vi "Module-error.vi"(6 "Error":T1=enum."Not implemented", 8 "error in (no error)":errorcluster, 9 "Overwrite?":bool, 10 "Additional message":string) -> (0 "error out":errorcluster)   [LabVIEW 2013, in "MaterialCharacterization.lvlib" / "MC-SM1000.lvclass"]
uses:
  MC-SM1000.lvclass
  Custom-errors.ctl
  <vilib>/Utility/error.llb/DialogType.ctl
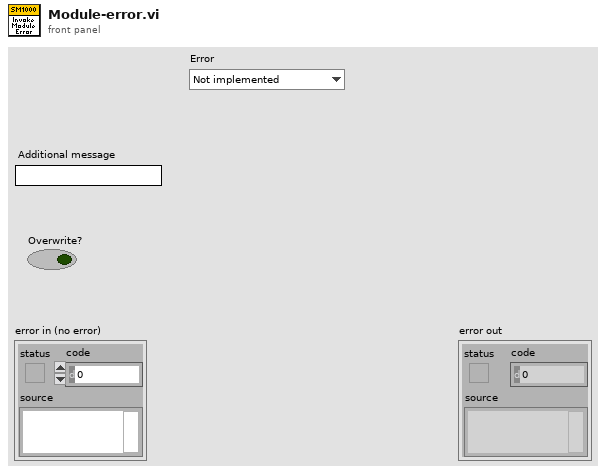
[diagram p1: front panel]
types:
  T1 = typedef "MaterialCharacterization.lvlib/MC-SM1000.lvclass/Custom-errors.ctl" = enum16{"No error", "Not implemented", "Command not recognized", "Invalid input", "No connection", "Timeout", "Resource not loaded"}
  T2 = typedef "DialogType.ctl" = u16
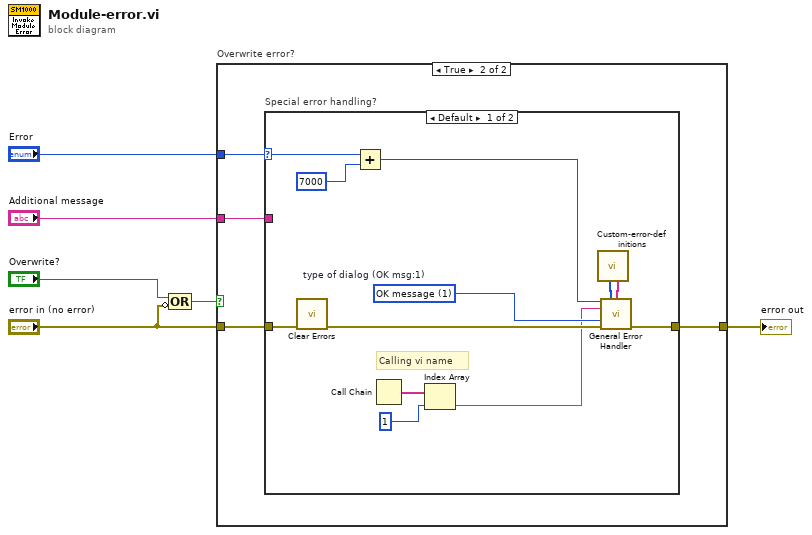
[diagram p0: block diagram]
diagram:
  n1 = Compound Arithmetic op=OR("Overwrite?", invert "error in (no error)") -> (w6:bool)
  n2 = case "Overwrite error?" shown="True" w6 {
    tunnel: [w7 w8] -> w4
    tunnel: "Error" -> [_ w11]
    tunnel: "Additional message" -> [_ w10]
    tunnel: "error in (no error)" -> [w7 w9]
    frame False {
    }
    frame True {
      n3 = case "Special error handling?" shown="Default" w11 {
        selector: w11 -> [w17 _]
        tunnel: [w20 w24] -> w8
        tunnel: w10 -> [_ _]
        tunnel: w9 -> [w21 w24]
        frame Default {
          w16 = T2 1 items=["no dialog", "OK message", "continue or stop message", "OK message + warnings", "continue/stop + warnings"]  # type of dialog (OK msg:1)
          # "Calling vi name"
          n4 = call <vilib>:"Clear Errors.vi"("error in (no error)"=w21) -> ("error out"=w15:errorcluster)  [unwired: 6 in]
          n5 = Add(x=w17, y=7000) -> (x+y=w19:i32)
          n6 = Call Chain() -> (call chain=w14:string[])
          n7 = Index Array(array=w14, index=1) -> (element=w12:string)
          n8 = call "Custom-error-definitions.vi"() -> ("Descriptions"=w23:string[], "Error codes"=w22:i32[])  [unwired: 10 in]
          n9 = call <vilib>:"General Error Handler.vi"("[error code] (0)"=w19, "[user-defined codes]"=w22, "[user-defined descriptions]"=w23, "[error source] (\" \")"=w12, "type of dialog (OK msg:1)"=w16, "error in (no error)"=w15) -> ("error out"=w20:errorcluster)  [unwired: 5 in, 4 out]
        }
        frame "No error" {
          # "No error."
        }
      }
    }
  }
  "error out" <- w4
